vi "connect.vi"(6 "wait for reply (T)":bool=TRUE, 8 "error in":errorcluster, 9 "connection":cluster{"ip":string, "port":u16, "timeout":i32}={"ip"="localhost", "port"=6379, "timeout"=1000}, 10 "flush":bool, 11 "Module ID":i32=-1) -> (0 "error out":errorcluster, 1 "timed out?":bool, 2 "status":cluster{"reply-to-ping":bool, "pong":bool})   [LabVIEW 2020, in "reporting-device.lvlib"]
doc: "connect to a redis instance\n_____\nCreated using DQMH Event Scripter 7.0.1.1316."
uses:
  reporting-device.lvlib
  connect Argument--cluster.ctl
  connect (Reply Payload)--cluster.ctl
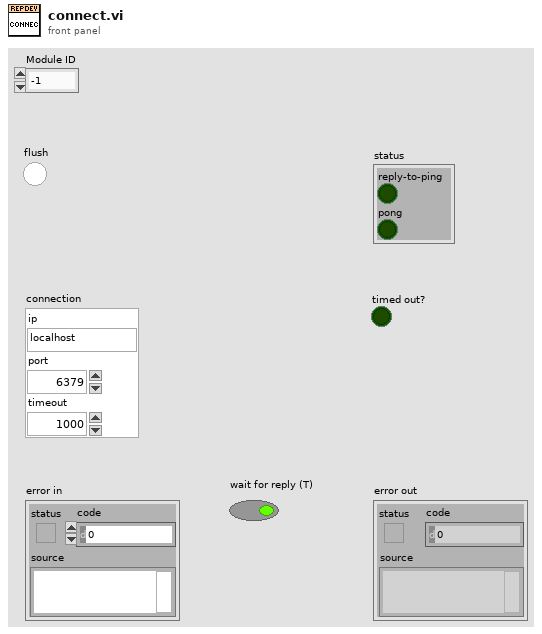
[diagram p1: front panel]
types:
  T1 = typedef "reporting-device.lvlib/connect Argument--cluster.ctl" = cluster{"Module ID":i32, "flush":bool, "connection":cluster{"ip":string, "port":u16, "timeout":i32}, "Wait Notifier":refnum<notifier>, "wait for reply":bool}
  T2 = typedef "reporting-device.lvlib/Request Events--cluster.ctl" = cluster{"Stop Module":refnum<user-event>, "Show Panel":refnum<user-event>, "Hide Panel":refnum<user-event>, "Show Diagram":refnum<user-event>, "Get Module Execution Status":refnum<user-event>, "connect":refnum<user-event>}
  T3 = typedef "reporting-device.lvlib/connect (Reply Payload)--cluster.ctl" = cluster{"Module ID":i32, "status":cluster{"reply-to-ping":bool, "pong":bool}, "error":errorcluster}
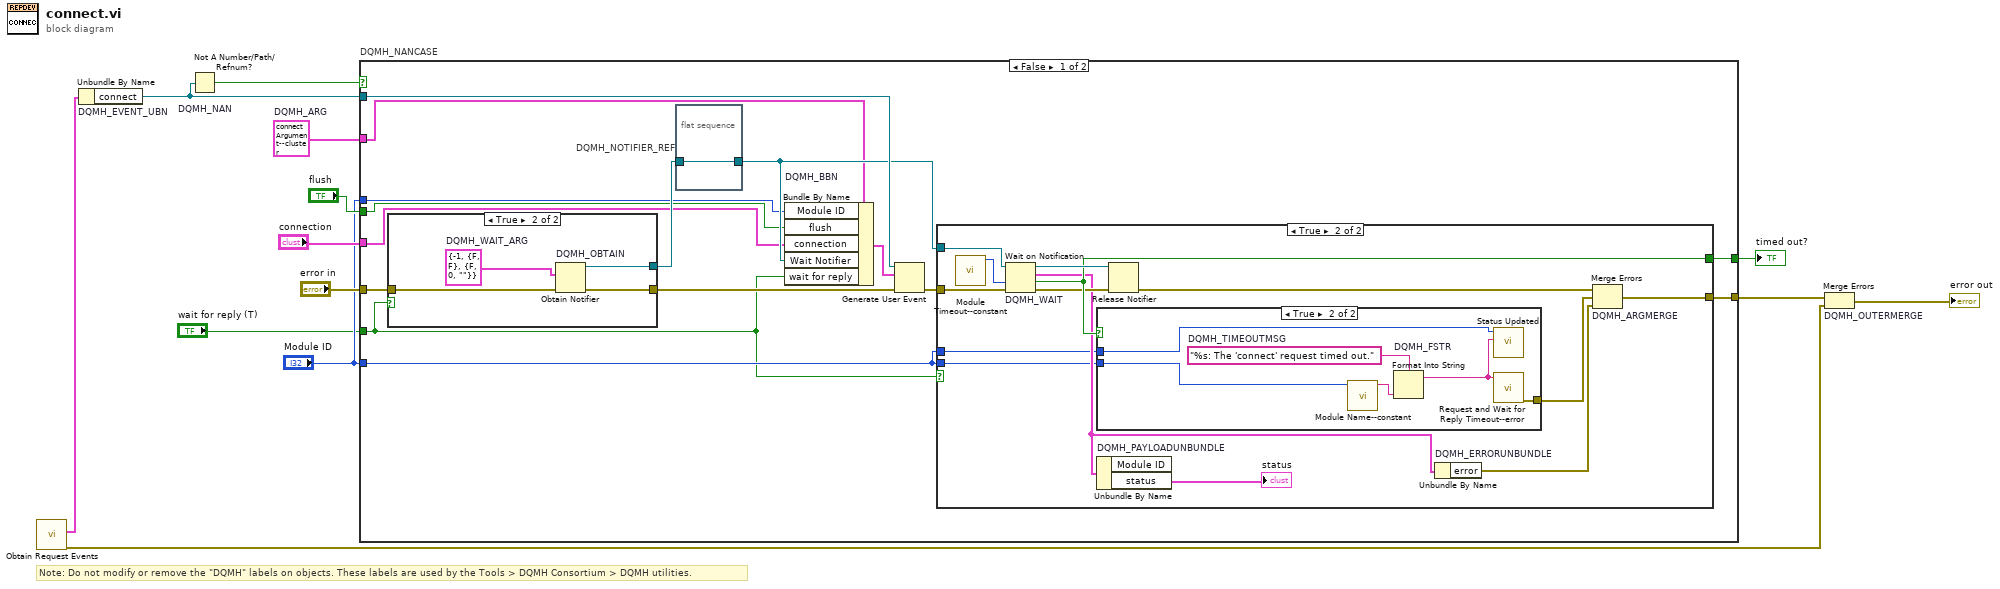
[diagram p0: block diagram]
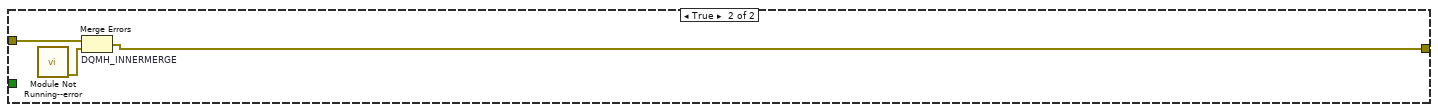
[diagram p5: hidden frame]
diagram:
  w7 = T1 {"Module ID"=-1, "flush"=FALSE, "connection"={"ip"="localhost", "port"=6379, "timeout"=1000}, "Wait Notifier"=refnum, "wait for reply"=FALSE}  # DQMH_ARG
  # "Note: Do not modify or remove the \"DQMH\" labels on objects. These labels are used by the Tools > DQMH Consortium > DQMH utilities."
  n1 = call "Obtain Request Events.vi"() -> ("error out"=w2:errorcluster, "reporting-device Request Events"=w1:T2)  [unwired: 10 in]
  n2 = Unbundle By Name "DQMH_EVENT_UBN"(w1) -> ("connect"=w11:refnum<user-event>)
  n3 = Not A Number/Path/Refnum? "DQMH_NAN"(number/path/refnum=w11) -> (NaN/Path/Refnum?=w10:bool)
  n4 = case "DQMH_NANCASE" shown="False" w10 {
    tunnel: "error in" -> [w28 w58]
    tunnel: w11 -> [w26 _]
    tunnel: [w23 w57] -> w8
    tunnel: [w24 _] -> w9
    tunnel: w7 -> [w19 _]
    tunnel: "Module ID" -> [w18 _]
    tunnel: "flush" -> [w17 _]
    tunnel: "connection" -> [w16 _]
    tunnel: "Module ID" -> [w15 _]
    tunnel: "wait for reply (T)" -> [w14 _]
    frame False {
      n5 = case shown="True" w14 {
        tunnel: w28 -> [w51 w55]
        tunnel: [w51 w54] -> w25
        tunnel: [_ w52] -> w21
        frame False {
        }
        frame True {
          w53 = T3 {"Module ID"=-1, "status"={"reply-to-ping"=FALSE, "pong"=FALSE}, "error"={"status"=FALSE, "code"=0, "source"=""}}  # DQMH_WAIT_ARG
          n6 = Obtain Notifier "DQMH_OBTAIN"(notification data type=w53, error in (no error)=w55) -> (notifier out=w52:refnum<notifier>, error out=w54:errorcluster)  [unwired: 2 in, 1 out]
        }
      }
      n7 = flat-sequence "DQMH_NOTIFIER_REF" {
        tunnel: w21 -> [w29]
        tunnel: [w29] -> w20
        frame #0 {
        }
      }
      n8 = Bundle By Name "DQMH_BBN"(cluster=w19, "Module ID"=w18, "flush"=w17, "connection"=w16, "Wait Notifier"=w20, "wait for reply"=w14) -> (w22:T1)
      n9 = Generate User Event(user event=w26, event data cluster=w22, error in=w25) -> (error out=w27:errorcluster)  [unwired: 1 in, 1 out]
      n10 = case shown="True" w14 {
        tunnel: w27 -> [w30 w44]
        tunnel: w20 -> [_ w43]
        tunnel: [_ w41] -> w24
        tunnel: [w30 w40] -> w23
        tunnel: w15 -> [_ w32]
        tunnel: w15 -> [_ w31]
        frame False {
        }
        frame True {
          n11 = call "Module Timeout--constant.vi"() -> ("Module Timeout"=w34:i32)  [unwired: 11 in]
          n12 = Wait on Notification "DQMH_WAIT"(notifier=w43, timeout in ms (-1)=w34, error in (no error)=w44) -> (notifier out=w42:refnum<notifier>, notification=w35:T3, timed out?=w41:bool, error out=w39:errorcluster)  [unwired: 1 in]
          n13 = case shown="True" w41 {
            tunnel: [_ w48] -> w36
            tunnel: w32 -> [_ w46]
            tunnel: w31 -> [_ w45]
            frame False {
            }
            frame True {
              w50 = "%s: The 'connect' request timed out."  # DQMH_TIMEOUTMSG
              n14 = call "Module Name--constant.vi"("Module ID"=w45) -> ("Module Name"=w47:string)  [unwired: 10 in]
              n15 = Format Into String "DQMH_FSTR"(format string=w50, w47) -> (resulting string=w49:string)  [unwired: 2 in, 1 out]
              n16 = call "Status Updated.vi"("Status"=w49, "Module ID"=w46) -> ()  [unwired: 9 in, 1 out]
              n17 = call "Request and Wait for Reply Timeout--error.vi"("Error Message"=w49) -> ("error out"=w48:errorcluster)  [unwired: 10 in]
            }
          }
          n18 = Unbundle By Name "DQMH_PAYLOADUNBUNDLE"(w35) -> ("status"=→"status":cluster{"reply-to-ping":bool, "pong":bool})  [unwired: 1 out]
          n19 = Release Notifier(notifier=w42, error in (no error)=w39) -> (error out=w38:errorcluster)  [unwired: 1 in, 2 out]
          n20 = Unbundle By Name "DQMH_ERRORUNBUNDLE"(w35) -> ("error"=w37:errorcluster)
          n21 = Merge Errors "DQMH_ARGMERGE"(w38, w36, w37) -> (w40:errorcluster)
        }
      }
    }
    frame True {
      n22 = call "Module Not Running--error.vi"() -> ("error out"=w56:errorcluster)  [unwired: 11 in]
      n23 = Merge Errors "DQMH_INNERMERGE"(w58, w56) -> (w57:errorcluster)
    }
  }
  "timed out?" <- w9
  n24 = Merge Errors "DQMH_OUTERMERGE"(w8, w2) -> (→"error out":errorcluster)
